vi "Operation Main.vi"(8 "error in (no error)":errorcluster, 11 "Task Factory In":refnum<class "Task Factory.lvclass">) -> (0 "error out":errorcluster, 3 "Task Factory Out":refnum<class "Task Factory.lvclass">)   [LabVIEW 2019, in "Task Factory.lvclass"]
uses:
  Task Factory.lvclass
  Task Factory MSG/Task Factory MSG.lvclass
  Ancestor Class/Message/Message.lvclass/Message.ctl
  Task Factory MSG/Task Factory MSG.lvclass/Task Factory MSG.ctl
  Ancestor Class/Message/Public Data/Read General CMD.vi
  Task Factory MSG/Public Data/Read Task Factory CMD.vi
  Ancestor Class/Message/Public Data/Read CMD Type.vi
  Ancestor Class/Message/Message.lvclass
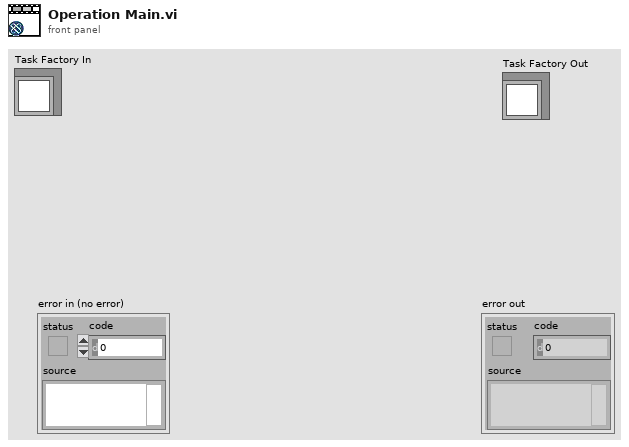
[diagram p1: front panel]
types:
  T1 = typedef "CMD Type.ctl" = enum16{"None", "General CMD", "1st CMD", "2nd CMD", "3rd CMD", "4th CMD", "5th CMD", "6th CMD", "7th CMD"}
  T2 = typedef "General CMD.ctl" = enum16{"None", "Stop", "Abort", "Running Task", "Running Batch Tasks", "Task Self Running", "Emergency Stop"}
  T3 = typedef "Task Factory CMD.ctl" = enum16{"None", "Generate Task"}
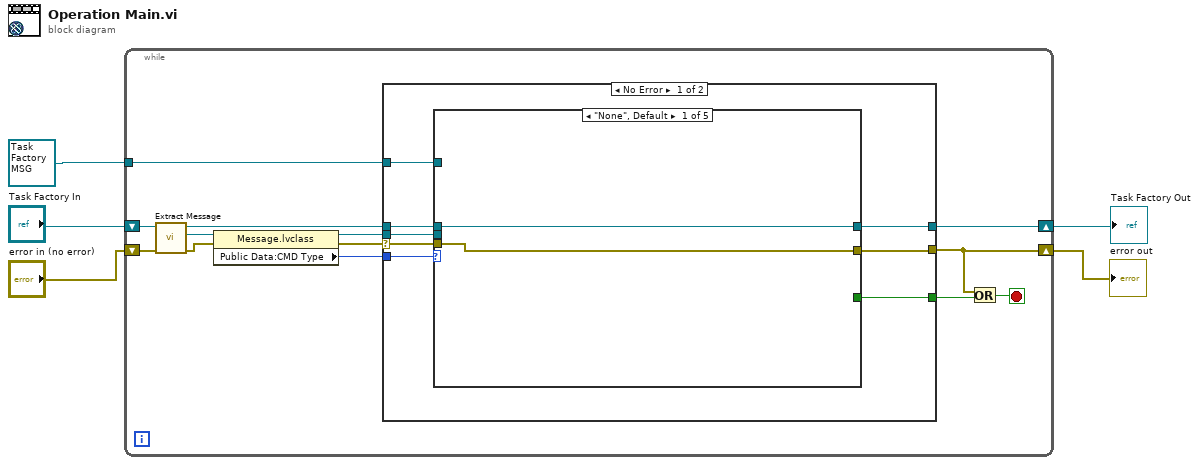
[diagram p0: block diagram]
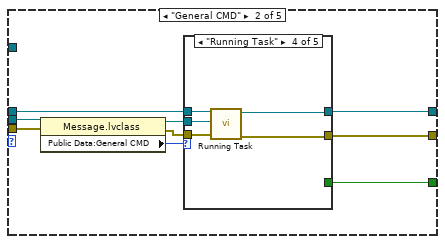
[diagram p2: hidden frame]
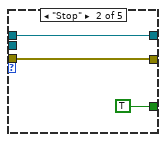
[diagram p4: hidden frame]
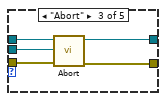
[diagram p5: hidden frame]
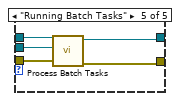
[diagram p6: hidden frame]
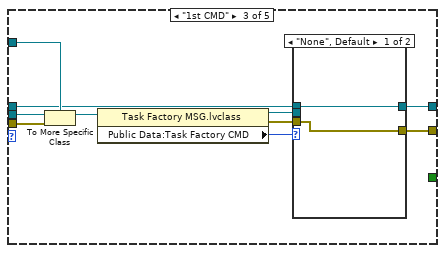
[diagram p7: hidden frame]
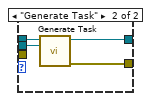
[diagram p8: hidden frame]
diagram:
  n1 = while {
    shift-right: [w7] -> w1
    shift-left: "Task Factory In" -> [w12]
    shift-right: [w14] -> w4
    shift-left: "error in (no error)" -> [w11]
    tunnel: refnum<class "Task Factory MSG.lvclass"> refnum ("Task Factory MSG.lvclass") -> [w13]
    stop <- w15 stop-if-true
    n2 = call-dynamic "Extract Message.vi"("error in (no error)"=w11, "System Actor in"=w12) -> ("error out"=w8:errorcluster, "Message Out"=w9:refnum<class "Message.lvclass">, "System Actor out"=w10:refnum<class "Task Factory.lvclass">)  [unwired: 6 in, 1 out]
    n3 = property class="Message.lvclass"(reference=w9, error in=w8) -> (reference out=w16:refnum<class "Message.lvclass">, error out=w17:errorcluster, "Public Data:CMD Type"=w18:T1)
    n4 = case shown="No Error" w17 {
      selector: w17 -> [w22 w78]
      tunnel: w18 -> [w26 _]
      tunnel: w10 -> [w24 w79]
      tunnel: [w23 w79] -> w7
      tunnel: w16 -> [w25 _]
      tunnel: [w20 w78] -> w14
      tunnel: w13 -> [w21 _]
      tunnel: [w19 _] -> w6
      frame No Error {
        n5 = case shown="\"None\", Default" w26 {
          tunnel: w25 -> [_ w37 w67 _ _]
          tunnel: w24 -> [w28 w34 w63 w75 w77]
          tunnel: [w28 w31 w61 w75 w77] -> w23
          tunnel: w22 -> [w27 w36 w66 w74 w76]
          tunnel: w21 -> [_ _ w65 _ _]
          tunnel: [w27 w30 w58 w74 w76] -> w20
          tunnel: [_ w29 _ _ _] -> w19
          frame "None", Default {
          }
          frame "General CMD" {
            n6 = property class="Message.lvclass"(reference=w37, error in=w36) -> (reference out=w33:refnum<class "Message.lvclass">, error out=w32:errorcluster, "Public Data:General CMD"=w35:T2)
            n7 = case shown="\"Running Task\"" w35 {
              tunnel: w34 -> [w39 w42 w47 w52 w57]
              tunnel: w33 -> [_ _ w46 w50 w56]
              tunnel: w32 -> [w38 w41 w45 w49 w55]
              tunnel: [w39 w42 w44 w51 w54] -> w31
              tunnel: [w38 w41 w43 w48 w53] -> w30
              tunnel: [_ TRUE _ _ _] -> w29
              frame "None", Default {
              }
              frame "Stop" {
              }
              frame "Abort" {
                n8 = call-dynamic "Abort.vi"("error in (no error)"=w45, "Message In"=w46, "System Actor in"=w47) -> ("error out"=w43:errorcluster, "System Actor out"=w44:refnum<class "Task Factory.lvclass">)  [unwired: 7 in]
              }
              frame "Running Task" {
                n9 = call-dynamic "Running Task.vi"("error in (no error)"=w49, "Message In"=w50, "System Actor in"=w52) -> ("error out"=w48:errorcluster, "System Actor out"=w51:refnum<class "Task Factory.lvclass">)  [unwired: 7 in]
              }
              frame "Running Batch Tasks" {
                n10 = call-dynamic "Process Batch Tasks.vi"("error in (no error)"=w55, "Message In"=w56, "System Actor in"=w57) -> ("error out"=w53:errorcluster, "System Actor out"=w54:refnum<class "Task Factory.lvclass">)  [unwired: 7 in]
              }
            }
          }
          frame "1st CMD" {
            n11 = To More Specific Class(target class=w65, reference=w67, error in=w66) -> (specific class reference=w64:refnum<class "Task Factory MSG.lvclass">)  [unwired: 1 out]
            n12 = property class="Task Factory MSG.lvclass"(reference=w64) -> (reference out=w60:refnum<class "Task Factory MSG.lvclass">, error out=w59:errorcluster, "Public Data:Task Factory CMD"=w62:T3)  [unwired: 1 in]
            n13 = case shown="\"None\", Default" w62 {
              tunnel: w63 -> [w69 w73]
              tunnel: [w69 w72] -> w61
              tunnel: w60 -> [_ w71]
              tunnel: w59 -> [w68 _]
              tunnel: [w68 w70] -> w58
              frame "None", Default {
              }
              frame "Generate Task" {
                n14 = call-dynamic "Generate Task.vi"("Task Factory MSG In"=w71, "Task Factory in"=w73) -> ("error out"=w70:errorcluster, "Task Factory out"=w72:refnum<class "Task Factory.lvclass">)  [unwired: 8 in]
              }
            }
          }
          frame "2nd CMD" {
          }
          frame "4th CMD" {
          }
        }
      }
      frame Error {
      }
    }
    n15 = Or(x=w14, y=w6) -> (x .or. y?=w15:bool)
  }
  "error out" <- w4
  "Task Factory Out" <- w1
